vi "Number of columns.vi"(8 "error in (no error)":errorcluster, 9 "Table Datas 2D":string[][](array[string]), 10 "Title 1D":string[](array[string]), 11 "columnWidth [ ]":sgl[](array[numeric])) -> (0 "error duplicate":errorcluster, 2 "numColumns":i32)   [LabVIEW 2012]
doc: "<B>ENGLISH</B>\nCreates a table with the given <B>numColumns</B> and the given <B>columnWidth [ ]</B>.\n\n<B>FRANÇAIS</B>\nCréation d'un tableau avec pour nombre de colonnes <B>numColumns</B> et dont les largeurs sont spécifiées par <B>columnWidth [ ]</B>.\n\nVersion 1.0\nDeveloped by Jean-Marc Simard\nCopyright © 2010, Exaprom Inc.\nAll rights reserved.\nLicense: BSD"
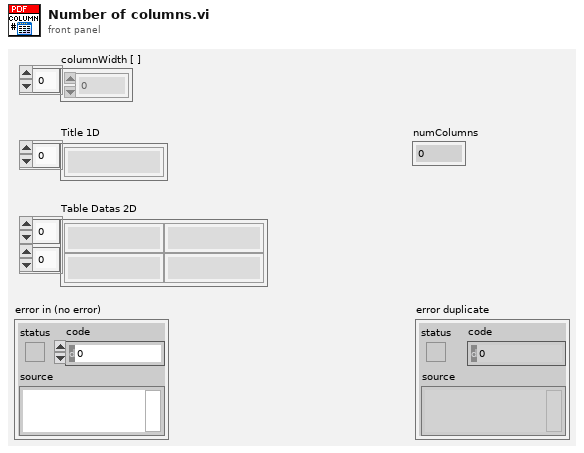
[diagram p1: front panel]
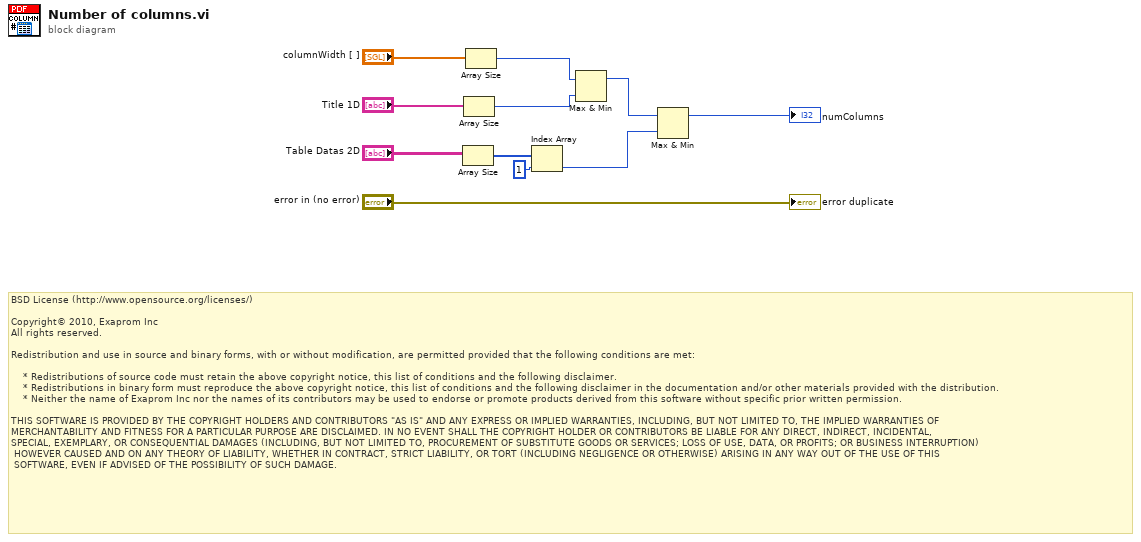
[diagram p0: block diagram]
diagram:
  # "BSD License (http://www.opensource.org/licenses/)\n\nCopyright© 2010, Exaprom Inc\nAll rights reserved.\n\nRedistribution and use in source and binary forms, with or without modification, are permitted provided that the following conditions are met:\n\n    * Redistributions of source code must retain the above copyright notice, this list of conditions and the following disclaimer.\n    * Redistributions in binary form must reproduce the above copyright notice, this list of conditions and the following disclaimer in the documentation and/or other materials provided with the distribution.\n    * Neither the name of Exaprom Inc nor the names of its contributors may be used to endorse or promote products derived from this software without specific prior written permission.\n\nTHIS SOFTWARE IS PROVIDED BY THE COPYRIGHT HOLDERS AND CONTRIBUTORS \"AS IS\" AND ANY EXPRESS OR IMPLIED WARRANTIES, INCLUDING, BUT NOT LIMITED TO, THE IMPLIED WARRANTIES OF \nMERCHANTABILITY AND FITNESS FOR A PARTICULAR PURPOSE ARE DISCLAIMED. IN NO EVENT SHALL THE COPYRIGHT HOLDER OR CONTRIBUTORS BE LIABLE FOR ANY DIRECT, INDIRECT, INCIDENTAL,\nSPECIAL, EXEMPLARY, OR CONSEQUENTIAL DAMAGES (INCLUDING, BUT NOT LIMITED TO, PROCUREMENT OF SUBSTITUTE GOODS OR SERVICES; LOSS OF USE, DATA, OR PROFITS; OR BUSINESS INTERRUPTION)\n HOWEVER CAUSED AND ON ANY THEORY OF LIABILITY, WHETHER IN CONTRACT, STRICT LIABILITY, OR TORT (INCLUDING NEGLIGENCE OR OTHERWISE) ARISING IN ANY WAY OUT OF THE USE OF THIS\n SOFTWARE, EVEN IF ADVISED OF THE POSSIBILITY OF SUCH DAMAGE."
  n1 = Array Size(array="Table Datas 2D") -> (size(s)=w6:i32[])
  n2 = Array Size(array="Title 1D") -> (size(s)=w3:i32)
  n3 = Array Size(array="columnWidth [ ]") -> (size(s)=w4:i32)
  n4 = Index Array(array=w6, index=1) -> (element=w1:i32)
  n5 = Max & Min(x=w4, y=w3) -> (max(x,y)=w2:i32)  [unwired: 1 out]
  n6 = Max & Min(x=w2, y=w1) -> (max(x,y)=→"numColumns":i32)  [unwired: 1 out]
  "error duplicate" <- "error in (no error)"
